vi "Device VI 1.0.vi"() -> ()   [LabVIEW 2017]
uses:
  <vilib>/Utility/error.llb/DialogType.ctl
  <vilib>/DAQmx/read.llb/DAQmx Read (Analog 1D Wfm NChan NSamp).vi
  <vilib>/DAQmx/create/channels.llb/DAQmx Create Channel (AI-Force-Bridge-Two-Point-Linear).vi
  <vilib>/DAQmx/configure/timing.llb/DAQmx Timing (Sample Clock).vi
  <vilib>/DAQmx/miscellaneous.llb/DAQmx Fill In Error Info.vi
  <vilib>/Utility/file.llb/Write Delimited Spreadsheet (DBL).vi
panel:
  in  "file path (dialog if empty)":path=path "C:/Users/Julio/Desktop/Device Data/Test.csv"
  in  "Samples per Loop":i32=100
  in  "Sample Rate":dbl=1000.0
  in  "Maximum Force":dbl=100.0
  in  "Minimum Force":dbl=-100.0
  in  "Bridge Information":T1={"Bridge Configuration"=10182, "Excitation Source"=10200, "Excitation Value"=2.5, "Nominal Resistance"=350.0} {"Excitation Source" items=["Internal"=10200, "External"=10167, "None"=10230]; "Bridge Configuration" items=["Full Bridge"=10182, "Half Bridge"=10187, "Quarter Bridge"=10270, "No Bridge"=10228]}
  in  "Physical Channels":tag="cDAQ2Mod1/ai0:cDAQ2Mod1/ai1"
  in  "Units (Force)":i32(ring)=15875 items=["Newtons"=15875, "Pounds"=15876, "kgf"=15877, "From Custom Scale"=10065]
  in  "Stop":bool
  out "Waveform Chart":waveform(dbl)[](graph)=[{"t0"=timestamp(3611924187.3904314 s since 1904-01-01), "dt"=0.001, "Y"=[7.7672034535118675, 7.7672034535118675, 7.7672034535118675, 7.7672034535118675, 7.7672034535118675, 7.7672034535118675, 7.7672034535118675, 7.7672034535118675, 7.7672034535118675, 7.7672034535118675, 7.7672034535118675, 7.7672034535118675, 7.7672034535118675, 7.7672034535118675, 7.7672034535118675, 7.7672034535118675, 7.7672034535118675, 7.7672034535118675, 7.7672034535118675, 7.7672034535118675, 7.7672034535118675, 7.7672034535118675, 7.7672034535118675, 7.7672034535118675, 7.7672034535118675, 7.7672034535118675, 7.7672034535118675, 7.7672034535118675, 7.7672034535118675, 7.7672034535118675, 7.7672034535118675, 7.7672034535118675, 7.7672034535118675, 7.7672034535118675, 7.7672034535118675, 7.7672034535118675, 7.7672034535118675, 7.7672034535118675, 7.7672034535118675, 7.7672034535118675, 7.7672034535118675, 7.7672034535118675, 7.7672034535118675, 7.7672034535118675, 7.7672034535118675, 7.7672034535118675, 7.7672034535118675, 7.7672034535118675, 7.7672034535118675, 7.7672034535118675, 7.7672034535118675, 7.7672034535118675, 7.7672034535118675, 7.7672034535118675, 7.7672034535118675, 7.7672034535118675, 7.7672034535118675, 7.7672034535118675, 7.7672034535118675, 7.7672034535118675, 7.7672034535118675, 7.7672034535118675, 7.7672034535118675, 7.7672034535118675, 7.7672034535118675, 7.7672034535118675, 7.7672034535118675, 7.7672034535118675, 7.7672034535118675, 7.7672034535118675, 7.7672034535118675, 7.7672034535118675, 7.7672034535118675, 7.7672034535118675, 7.7672034535118675, 7.7672034535118675, 7.7672034535118675, 7.7672034535118675, 7.7672034535118675, 7.7672034535118675, 7.7672034535118675, 7.7672034535118675, 7.7672034535118675, 7.7672034535118675, 7.7672034535118675, 7.7672034535118675, 7.7672034535118675, 7.7672034535118675, 7.7672034535118675, 7.7672034535118675, 7.7672034535118675, 7.7672034535118675, 7.7672034535118675, 7.7672034535118675, 7.7672034535118675, 7.7672034535118675, 7.7672034535118675, 7.7672034535118675, 7.7672034535118675, 7.7672034535118675], "attributes"=variant("NI_ChannelName"=variant(string "cDAQ2Mod1/ai0"), "NI_UnitDescription"=variant(string "Newtons"))}, {"t0"=timestamp(3611924187.3904314 s since 1904-01-01), "dt"=0.001, "Y"=[-1.2515185680867968, -1.2515185680867968, -1.2515185680867968, -1.2515185680867968, -1.2515185680867968, -1.2515185680867968, -1.2515185680867968, -1.2515185680867968, -1.2515185680867968, -1.2515185680867968, -1.2515185680867968, -1.2515185680867968, -1.2515185680867968, -1.2515185680867968, -1.2515185680867968, -1.2515185680867968, -1.2515185680867968, -1.2515185680867968, -1.2515185680867968, -1.2515185680867968, -1.2515185680867968, -1.2515185680867968, -1.2515185680867968, -1.2515185680867968, -1.2515185680867968, -1.2515185680867968, -1.2515185680867968, -1.2515185680867968, -1.2515185680867968, -1.2515185680867968, -1.2515185680867968, -1.2515185680867968, -1.2515185680867968, -1.2515185680867968, -1.2515185680867968, -1.2515185680867968, -1.2515185680867968, -1.2515185680867968, -1.2515185680867968, -1.2515185680867968, -1.2515185680867968, -1.2515185680867968, -1.2515185680867968, -1.2515185680867968, -1.2515185680867968, -1.2515185680867968, -1.2515185680867968, -1.2515185680867968, -1.2515185680867968, -1.2515185680867968, -1.2515185680867968, -1.2515185680867968, -1.2515185680867968, -1.2515185680867968, -1.2515185680867968, -1.2515185680867968, -1.2515185680867968, -1.2515185680867968, -1.2515185680867968, -1.2515185680867968, -1.2515185680867968, -1.2515185680867968, -1.2515185680867968, -1.2515185680867968, -1.2515185680867968, -1.2515185680867968, -1.2515185680867968, -1.2515185680867968, -1.2515185680867968, -1.2515185680867968, -1.2515185680867968, -1.2515185680867968, -1.2515185680867968, -1.2515185680867968, -1.2515185680867968, -1.2515185680867968, -1.2515185680867968, -1.2515185680867968, -1.2515185680867968, -1.2515185680867968, -1.2515185680867968, -1.2515185680867968, -1.2515185680867968, -1.2515185680867968, -1.2515185680867968, -1.2515185680867968, -1.2515185680867968, -1.2515185680867968, -1.2515185680867968, -1.2515185680867968, -1.2515185680867968, -1.2515185680867968, -1.2515185680867968, -1.2515185680867968, -1.2515185680867968, -1.2515185680867968, -1.2515185680867968, -1.2515185680867968, -1.2515185680867968, -1.2515185680867968], "attributes"=variant("NI_ChannelName"=variant(string "cDAQ2Mod1/ai1"), "NI_UnitDescription"=variant(string "Newtons"))}]
  # "Settings"
  # "Trigger Settings"
  # "2 Channel Data"
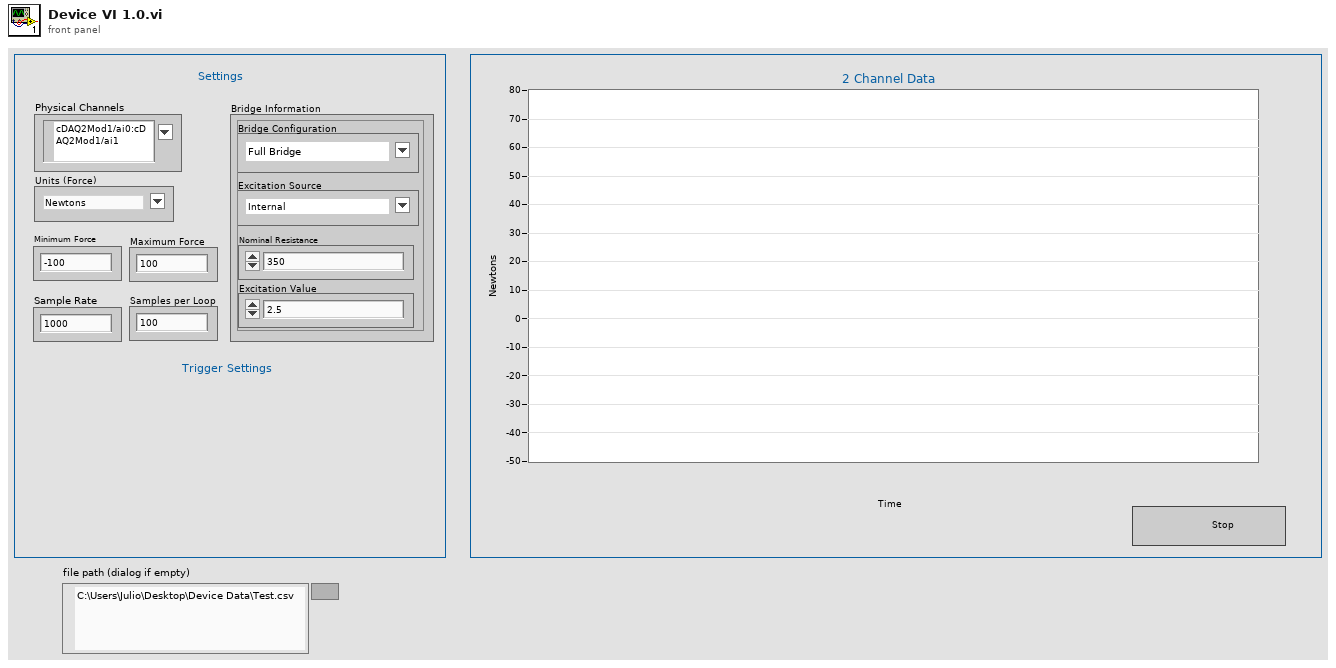
[diagram p1: front panel]
types:
  T1 = cluster{"Bridge Configuration":i32, "Excitation Source":i32, "Excitation Value":dbl, "Nominal Resistance":dbl}
  T2 = typedef "DialogType.ctl" = u16
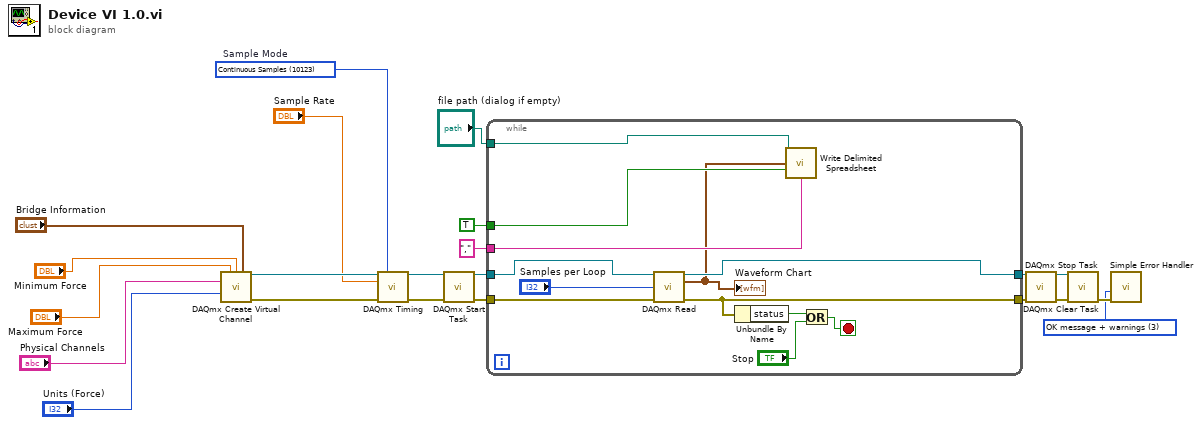
[diagram p0: block diagram]
diagram:
  w11 = T2 3 items=["no dialog", "OK message", "continue or stop message", "OK message + warnings", "continue/stop + warnings"] ("type of dialog (OK msg:1)")
  w20 = 10123 items=["Finite Samples"=10178, "Continuous Samples"=10123, "Hardware Timed Single Point"=12522]  # Sample Mode
  n1 = call-poly <vilib>:"DAQmx Create Virtual Channel.vi"("maximum value"="Maximum Force", "minimum value"="Minimum Force", "bridge information"="Bridge Information", "physical channels"="Physical Channels", "units"="Units (Force)") -> ("task out"=w22:refnum<k21>, "error out"=w21:errorcluster)  [unwired: 9 in]
  n2 = call-poly <vilib>:"DAQmx Timing.vi"("task/channels in"=w22, "sample mode"=w20, "rate"="Sample Rate", "error in"=w21) -> ("task out"=w18:refnum<k21>, "error out"=w17:errorcluster)  [unwired: 10 in]
  n3 = call <vilib>:"DAQmx Start Task.vi"("task/channels in"=w18, "error in"=w17) -> ("task out"=w10:refnum<k21>, "error out"=w9:errorcluster)  [unwired: 12 in]
  n4 = while {
    tunnel: w10 -> [w27]
    tunnel: [w32] -> w14
    tunnel: [w33] -> w15
    tunnel: w9 -> [w28]
    tunnel: "file path (dialog if empty)" -> [w26]
    tunnel: TRUE -> [w25]
    tunnel: "," ("delimiter (\\t)") -> [w24]
    stop <- w34 stop-if-true
    n5 = call-poly <vilib>:"DAQmx Read.vi"("task/channels in"=w27, "number of samples per channel"="Samples per Loop", "error in"=w28) -> ("task out"=w33:refnum<k21>, "data"=w23:waveform(dbl)[], "error out"=w32:errorcluster)  [unwired: 10 in]
    "Waveform Chart" <- w23
    n6 = Unbundle By Name(w32) -> ("status"=w31:bool)
    n7 = call-poly <vilib>:"Write Delimited Spreadsheet.vi"("file path (dialog if empty)"=w26, "1D data"=w23, "append to file? (new file:F)"=w25, "delimiter (\\t)"=w24) -> ()  [unwired: 10 in, 2 out]
    n8 = Or(x=w31, y="Stop") -> (x .or. y?=w34:bool)
  }
  n9 = call <vilib>:"DAQmx Stop Task.vi"("task/channels in"=w15, "error in"=w14) -> ("task out"=w13:refnum<k21>, "error out"=w12:errorcluster)  [unwired: 12 in]
  n10 = call <vilib>:"DAQmx Clear Task.vi"("task in"=w13, "error in"=w12) -> ("error out"=w16:errorcluster)  [unwired: 13 in]
  n11 = call <vilib>:"Simple Error Handler.vi"("type of dialog (OK msg:1)"=w11, "error in (no error)"=w16) -> ()  [unwired: 3 in, 5 out]
